vi "sub_strain-offset.vi"(8 "error in":errorcluster) -> (0 "error out":errorcluster)   [LabVIEW 2013]
uses:
  ctl/strain_ctl.ctl
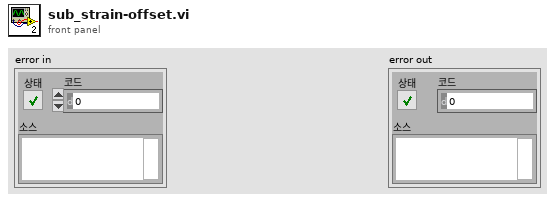
[diagram p1: front panel]
types:
  T1 = typedef "strain_ctl.ctl" = enum16{"config", "start", "read", "close"}
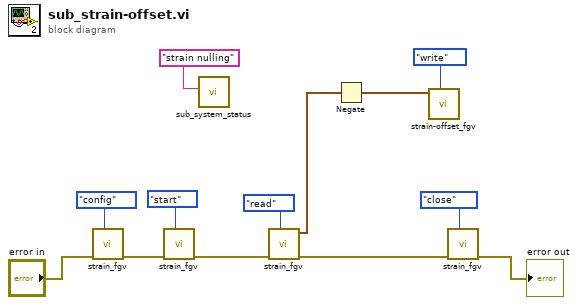
[diagram p0: block diagram]
diagram:
  n1 = call "strain_fgv.vi"("cmd"=strain_ctl."config", "error in"="error in") -> ("error out"=w9:errorcluster)  [unwired: 8 in, 1 out]
  n2 = call "strain_fgv.vi"("cmd"=strain_ctl."start", "error in"=w9) -> ("error out"=w8:errorcluster)  [unwired: 8 in, 1 out]
  n3 = call "sub_system_status.vi"("String in"="strain nulling") -> ()  [unwired: 10 in, 1 out]
  n4 = call "strain_fgv.vi"("cmd"=strain_ctl."read", "error in"=w8) -> ("error out"=w6:errorcluster, "data"=w10:waveform(dbl)[])  [unwired: 8 in]
  n5 = Negate(x=w10) -> (-x=w2:waveform(dbl)[])
  n6 = call "strain-offset_fgv.vi"("cmd"=enum16{"ini", "write", "read"}."write", "data"=w2) -> ()  [unwired: 9 in, 1 out]
  n7 = call "strain_fgv.vi"("cmd"=strain_ctl."close", "error in"=w6) -> ("error out"=→"error out":errorcluster)  [unwired: 8 in, 1 out]
